vi "to_json.vi"(8 "error in":errorcluster, 11 "containerized in":refnum<class "containerized.lvclass">) -> (0 "error out":errorcluster, 2 "json":string, 3 "containerized out":refnum<class "containerized.lvclass">, 4 "Not Default":bool)   [LabVIEW 2020, in "datasources.lvlib" / "containerized.lvclass"]
uses:
  containerized.lvclass
  containerized.lvclass/containerized.ctl
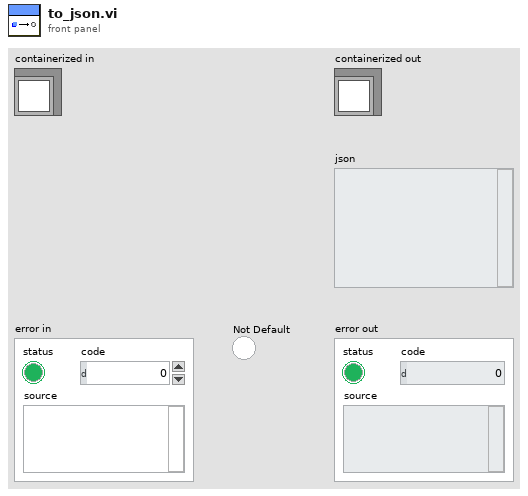
[diagram p1: front panel]
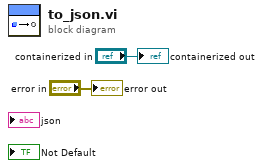
[diagram p0: block diagram]
diagram:
  "containerized out" <- "containerized in"
  "error out" <- "error in"
